vi "function generator.vi"() -> ()   [LabVIEW 2009]
uses:
  <vilib>/rvi/DataTransferAndStorage/Container/XNode/niFpgaContainer.xnode
  <vilib>/rvi/interface/RandomDataEmulation/niFpgaRandomDataHandleErrors.vi
  <vilib>/rvi/interface/RandomDataEmulation/nirviRandomDataFPGAFIFO.vi
  <vilib>/rvi/DataTransferAndStorage/Container/Common/niFpgaContainerMethod.ctl
  <vilib>/rvi/DataTransferAndStorage/Container/Common/niFpgaTransferTypeControl.ctl
  Instance           3 24Saved   Streamlined FPGA .vi
  Instance           4 24Saved   Streamlined FPGA .vi
  <vilib>/eio/EIONode/EIONode.xnode
  <vilib>/rvi/eio/nirviEIOImplementation/nirviEIOImplementation.xnode
  <vilib>/rvi/eio/common/nirviEmuTemplateMethod_noerrors.vi
  <vilib>/rvi/eio/common/nirviEmuClasses.ctl
  Instance           5 24Saved   Streamlined FPGA .vi
panel:
  out "sort pulse":i16
  out "Full 2":bool
  in  "Gain 1":i16(slide) scale=-32767.0..32767.0
  in  "Gain 2":i16(slide) scale=-32767.0..32767.0
  in  "Gain 3":i16(slide) scale=-32767.0..32767.0
  in  "Gain 4":i16(slide) scale=-32767.0..32767.0
  in  "amplitude":i16
  in  "1/Frequency \n(ticks)":u32
  in  "Burst \nCycles":i32
  in  "delay [us]":u32=20 min=1 max=8000
  # "Acquisition and Detection"
  # "FP and Sorting Parameters"
  # "Sorting Pulse\nGenerator"
  # "Events"
  # "PMT Controls"
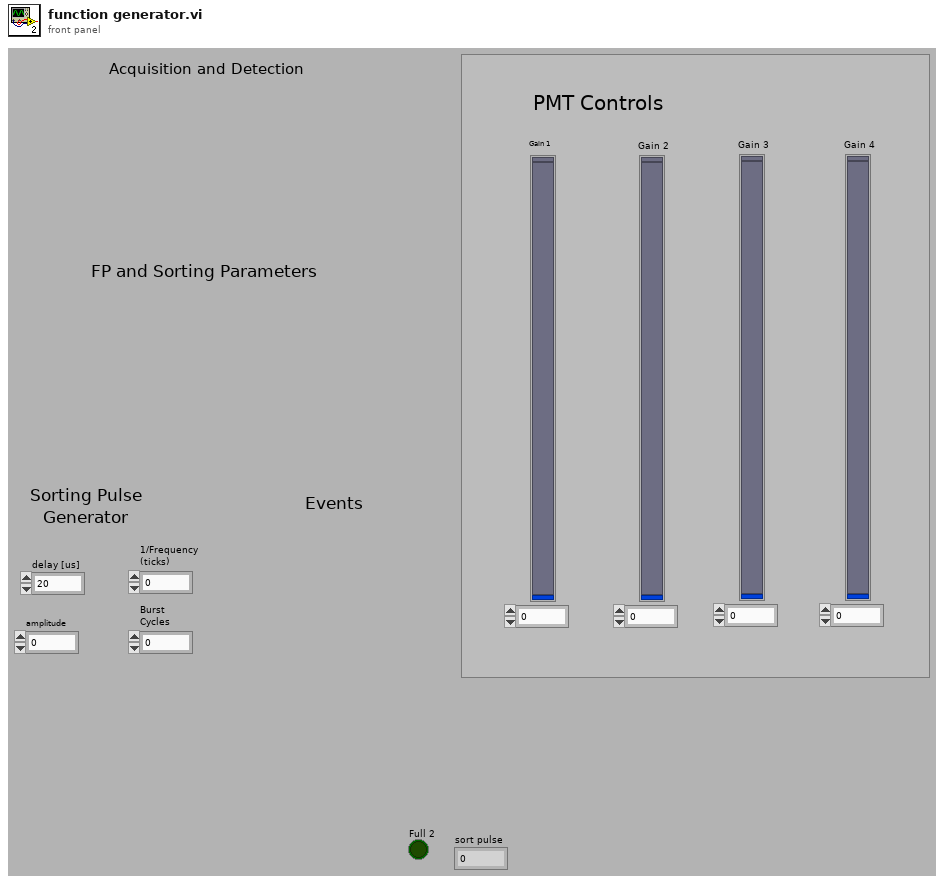
[diagram p1: front panel]
types:
  T1 = typedef "niFpgaContainerMethod.ctl" = enum16{"Write", "Read", "Clear", "Get Number of Elements to Write", "Get Number of Elements to Read", "Enable", "Disable", "Flush and Disable", "Get Stream State"}
  T2 = typedef "niFpgaTransferTypeControl.ctl" = enum16{"Target-Scoped", "Host to Target - DMA", "Target to Host - DMA", "Peer to Peer Reader", "Peer to Peer Writer", "Bidirectional"}
  T3 = typedef "nirviEmuClasses.ctl" = enum16{"IO Read", "IO Write", "Method", "Property Read", "Property Write"}
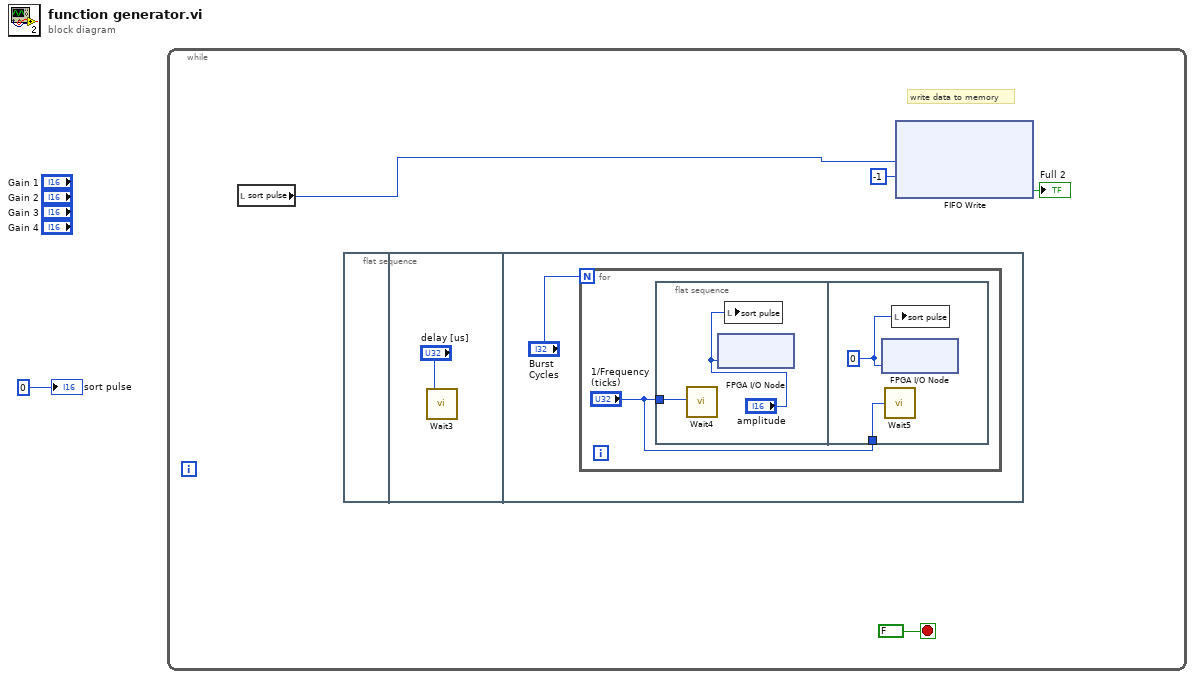
[diagram p0: block diagram]
diagram:
  n1 = while {
    stop <- FALSE stop-if-true
    # "write data to memory"
    n2 = local read "sort pulse"() -> (w4:i16)
    n3 = flat-sequence {
      frame #0 {
      }
      frame #1 {
        n4 = call "Wait3"("Count(uSec)"="delay [us]") -> ()  [unwired: 1 out]
      }
      frame #2 {
        n5 = for {
          N: "Burst \nCycles" -> [_]
          n6 = flat-sequence {
            tunnel: "1/Frequency \n(ticks)" -> [w35]
            tunnel: "1/Frequency \n(ticks)" -> [w48]
            frame #0 {
              n7 = call "Wait4"("Count(Ticks)"=w35) -> ()  [unwired: 1 out]
              n8 = xnode "FPGA I/O Node"("AO4"="amplitude") -> ()  [unwired: 1 in, 1 out]
              n9 = local write "sort pulse"("amplitude") -> ()
            }
            frame #1 {
              w47 = i16 0 ("sort pulse")
              n10 = xnode "FPGA I/O Node"("AO4"=w47) -> ()  [unwired: 1 in, 1 out]
              n11 = call "Wait5"("Count(Ticks)"=w48) -> ()  [unwired: 1 out]
              n12 = local write "sort pulse"(w47) -> ()
            }
          }
        }
      }
    }
    n13 = xnode ("FIFO Write")("Element"=w4, "Timeout"=-1) -> ("Timed Out?"=→"Full 2":bool)  [unwired: 1 in, 1 out]
  }
  "sort pulse" <- i16 0 ("event counter")
